vi "Client.vi"() -> ()   [LabVIEW 2020]
doc: "The queue refnums only work for communication within a single LabVIEW application instance. They cannot be used for communicating with another app instance on the same machine nor on any remote machines. This example shows how to combine queues with TCP (or any other communications protocol) to be able to have networked queues. The example is written using the address \"localhost\" so that both the client and server VIs may be on the same machine. If you want to actually use the example on separate machines, put the appropriate IP addresses into the constants on the block diagrams."
uses:
  Queue Type.ctl
panel:
  out "Receiver 2":T1
  out "Receiver 1":T1
  in  "stop":bool
  # "Run this VI first, then start Server.vi."
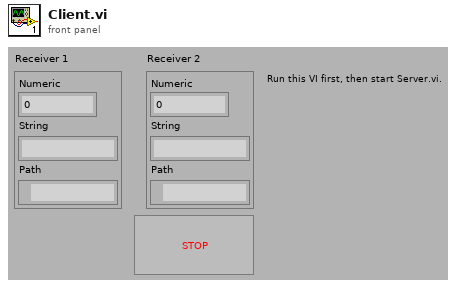
[diagram p1: front panel]
types:
  T1 = typedef "Queue Type.ctl" = cluster{"Numeric":dbl, "String":string, "Path":path}
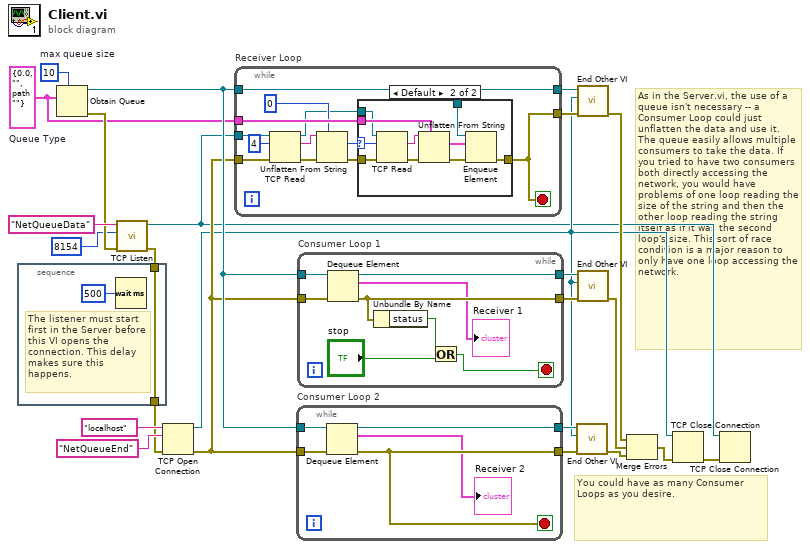
[diagram p0: block diagram]
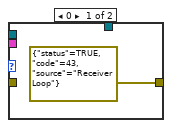
[diagram p2: hidden frame]
diagram:
  w1 = 10  # max queue size
  w4 = T1 {"Numeric"=0.0, "String"="", "Path"=path ""}  # Queue Type
  # "As in the Server.vi, the use of a queue isn't necessary -- a Consumer Loop could just unflatten the data and use it. The queue easily allows multiple consumers to take the data. If you tried to have two consumers both directly accessing the network, you would have problems of one loop reading the size of the string and then the other loop reading the string itself as if it was the second loop's size. This sort of race condition is a major reason to only have one loop accessing the network."
  # "You could have as many Consumer Loops as you desire."
  n1 = Obtain Queue(max queue size (-1, unlimited)=w1, element data type=w4) -> (queue out=w12:refnum<queue>, error out=w23:errorcluster)  [unwired: 2 in, 2 out]
  n2 = call <vilib>:"TCP Listen.vi"("error in (no error)"=w23, "port"=u16 8154, "service name"="NetQueueData" ("address")) -> ("error out"=w2:errorcluster, "connection ID"=w5:refnum<k5>)  [unwired: 1 in, 6 out]
  n3 = stacked-sequence {
    tunnel: [w26] -> w3
    tunnel: w2 -> [w26]
    frame #0 {
      # "The listener must start first in the Server before this VI opens the connection. This delay makes sure this happens."
      n4 = Wait (ms)(milliseconds to wait=u32 500) -> ()  [unwired: 1 out]
    }
  }
  n5 = TCP Open Connection(address="localhost", remote port or service name="NetQueueEnd" ("address"), error in (no error)=w3) -> (connection ID=w6:refnum<k5>, error out=w11:errorcluster)  [unwired: 2 out]
  n6 = while "Receiver Loop" {
    tunnel: w12 -> [w35]
    tunnel: w11 -> [w37]
    tunnel: w5 -> [w38]
    tunnel: [w35] -> w17
    tunnel: [w36] -> w16
    tunnel: w4 -> [w34]
    stop <- w36 stop-if-true
    n7 = TCP Read(connection ID=w38, bytes to read=4, error in (no error)=w37) -> (connection ID out=w27:refnum<k5>, data out=w30:string, error out=w32:errorcluster)  [unwired: 2 out]
    n8 = Unflatten From String(type=0, binary string=w30, error in (no error)=w32) -> (value=w28:i32, error out=w31:errorcluster)  [unwired: 3 out]
    n9 = case shown="Default" w28 {
      selector: w28 -> [_ w41]
      tunnel: w34 -> [_ w49]
      tunnel: w31 -> [_ w42]
      tunnel: w35 -> [_ w48]
      tunnel: [errorcluster {"status"=TRUE, "code"=43, "source"="Receiver Loop"} ("error out") w45] -> w36
      tunnel: w27 -> [_ w40]
      frame 0 {
      }
      frame Default {
        n10 = TCP Read(connection ID=w40, bytes to read=w41, error in (no error)=w42) -> (data out=w43:string, error out=w44:errorcluster)  [unwired: 3 out]
        n11 = Unflatten From String(type=w49, binary string=w43, error in (no error)=w44) -> (value=w47:T1, error out=w46:errorcluster)  [unwired: 3 out]
        n12 = Enqueue Element(queue=w48, element=w47, error in (no error)=w46) -> (error out=w45:errorcluster)  [unwired: 3 out]
      }
    }
  }
  n13 = while "Consumer Loop 2" {
    tunnel: w12 -> [w54]
    tunnel: w11 -> [w53]
    tunnel: [w52] -> w9
    tunnel: [w51] -> w10
    stop <- w51 stop-if-true
    n14 = Dequeue Element(queue=w54, error in (no error)=w53) -> (queue out=w52:refnum<queue>, element=→"Receiver 2":T1, error out=w51:errorcluster)  [unwired: 2 out]
  }
  n15 = while "Consumer Loop 1" {
    tunnel: w12 -> [w62]
    tunnel: w11 -> [w61]
    tunnel: [w57] -> w15
    tunnel: [w56] -> w14
    stop <- w58 stop-if-true
    n16 = Dequeue Element(queue=w62, error in (no error)=w61) -> (queue out=w57:refnum<queue>, element=→"Receiver 1":T1, error out=w56:errorcluster)  [unwired: 2 out]
    n17 = Unbundle By Name(w56) -> ("status"=w60:bool)
    n18 = Or(x=w60, y="stop") -> (x .or. y?=w58:bool)
  }
  n19 = call "End Other VI.vi"("error in (no error)"=w10, "TCP Connection"=w6, "queue in"=w9) -> ("error out"=w13:errorcluster)  [unwired: 8 out]
  n20 = call "End Other VI.vi"("error in (no error)"=w16, "TCP Connection"=w6, "queue in"=w17) -> ("error out"=w21:errorcluster)  [unwired: 8 out]
  n21 = call "End Other VI.vi"("error in (no error)"=w14, "TCP Connection"=w6, "queue in"=w15) -> ("error out"=w20:errorcluster)  [unwired: 8 out]
  n22 = Merge Errors(w21, w20, w13) -> (w19:errorcluster)
  n23 = TCP Close Connection(connection ID=w6, error in (no error)=w19) -> (error out=w18:errorcluster)  [unwired: 2 out]
  n24 = TCP Close Connection(connection ID=w5, error in (no error)=w18) -> ()  [unwired: 3 out]
